vi "RT-PC Main.vi"() -> ()   [LabVIEW 2016]
panel:
  out "received message":string
  out "success":bool
  in  "[ESC]":bool
  in  "my name":string="name"
  in  "ping":bool
  in  "listening port":u16=50001
  in  "destination IP address":string
  out "my primary IP address":string
  out "my available IP addresses":string[](array[string])
  out "number of addresses":i32
  # "TCP ping"
  # "restart VI after changing\nlistening port number"
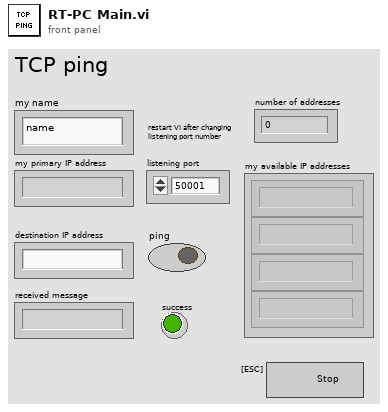
[diagram p1: front panel]
types:
  T1 = enum16{"Standard", "Buffered", "CRLF", "Immediate"}
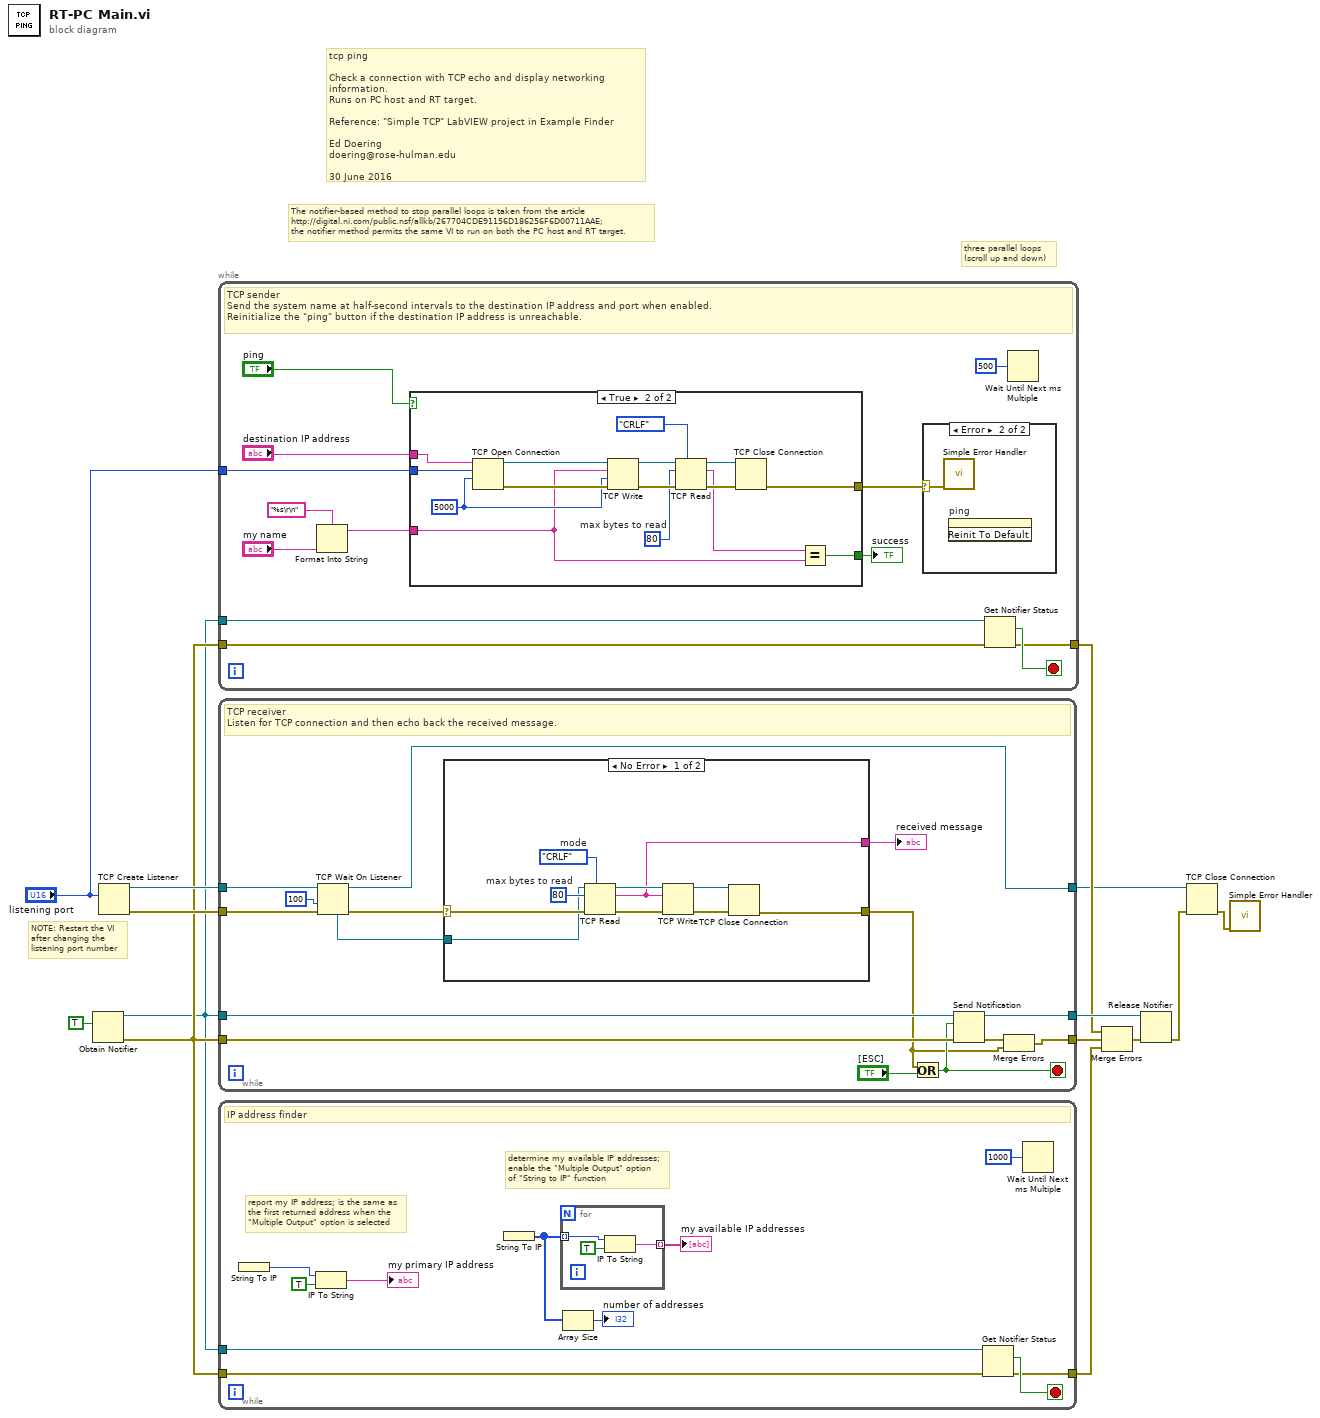
[diagram p0: block diagram]
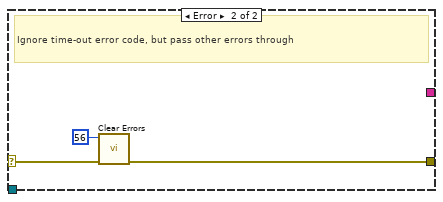
[diagram p2: hidden frame]
diagram:
  # "NOTE: Restart the VI\nafter changing the\nlistening port number"
  # "The notifier-based method to stop parallel loops is taken from the article\nhttp://digital.ni.com/public.nsf/allkb/267704CDE91156D186256F6D00711AAE;\nthe notifier method permits the same VI to run on both the PC host and RT target."
  # "three parallel loops\n(scroll up and down)"
  # "tcp ping\n\nCheck a connection with TCP echo and display networking information.\nRuns on PC host and RT target.\n\nReference: \"Simple TCP\" LabVIEW project in Example Finder \n\nEd Doering\ndoering@rose-hulman.edu\n\n30 June 2016"
  n1 = Obtain Notifier(notification data type=TRUE ("dot notation? (F)")) -> (notifier out=w4:refnum<notifier>, error out=w5:errorcluster)  [unwired: 3 in, 1 out]
  n2 = TCP Create Listener(10:"listening port") -> (0:w14:errorcluster, 3:w13:refnum<k5>)  [unwired: 4 in, 1 out]
  n3 = while {
    tunnel: w5 -> [w21]
    tunnel: w4 -> [w20]
    tunnel: [w18] -> w3
    tunnel: "listening port" -> [w15]
    stop <- w19 stop-if-true
    # "TCP sender\nSend the system name at half-second intervals to the destination IP address and port when enabled.\nReinitialize the \"ping\" button if the destination IP address is unreachable."
    n4 = Format Into String "Format Into String"(format string="%s\r\n", "my name") -> (resulting string=w24:string)  [unwired: 2 in, 1 out]
    n5 = case shown="True" "ping" {
      tunnel: [_ w33] -> w22
      tunnel: w24 -> [_ w32]
      tunnel: "destination IP address" -> [_ w43]
      tunnel: w15 -> [_ w42]
      tunnel: [_ w29] -> w16
      frame False {
      }
      frame True {
        w36 = 80  # max bytes to read
        w39 = 5000 ("timeout ms (60000)")
        n6 = TCP Open Connection(address=w43, remote port or service name=w42, timeout ms (60000)=w39) -> (connection ID=w40:refnum<k5>, error out=w41:errorcluster)  [unwired: 2 in]
        n7 = TCP Write(connection ID=w40, data in=w32, error in (no error)=w41, 9:w39) -> (connection ID out=w38:refnum<k5>, error out=w37:errorcluster)  [unwired: 1 out]
        n8 = TCP Read(connection ID=w38, bytes to read=w36, error in (no error)=w37, 7:T1."CRLF" ("mode (standard)")) -> (connection ID out=w34:refnum<k5>, data out=w30:string, error out=w35:errorcluster)  [unwired: 1 in]
        n9 = TCP Close Connection(connection ID=w34, error in (no error)=w35) -> (error out=w33:errorcluster)  [unwired: 1 in, 1 out]
        n10 = Equal?(x=w30, y=w32) -> (x = y?=w29:bool)
      }
    }
    "success" <- w16
    n11 = case shown="Error" w22 {
      selector: w22 -> [_ w28]
      frame No Error {
      }
      frame Error {
        n12 = call <vilib>:"Simple Error Handler.vi"("error in (no error)"=w28) -> ()  [unwired: 4 in, 5 out]
        n13 = invoke on="ping" class="Bool (strict)" method="Reinit To Default"() -> ()  [unwired: 3 in, 3 out]
      }
    }
    n14 = Get Notifier Status(notifier=w20, error in (no error)=w21) -> (current notification=w19:bool, error out=w18:errorcluster)  [unwired: 3 out]
    n15 = Wait Until Next ms Multiple(millisecond multiple=u32 500) -> ()  [unwired: 1 out]
  }
  n16 = while {
    tunnel: w13 -> [w58]
    tunnel: [w54] -> w1
    tunnel: w14 -> [w57]
    tunnel: w4 -> [w53]
    tunnel: w5 -> [w52]
    tunnel: [w46] -> w6
    tunnel: [w49] -> w11
    stop <- w50 stop-if-true
    # "TCP receiver\nListen for TCP connection and then echo back the received message."
    n17 = TCP Wait On Listener(8:w57, 9:100 ("timeout ms (25000)"), 11:w58) -> (0:w56:errorcluster, 3:w54:refnum<k5>, 4:w45:refnum<k5>)  [unwired: 1 in, 2 out]
    n18 = case shown="No Error" w56 {
      selector: w56 -> [w62 w71]
      tunnel: [w61 w70] -> w47
      tunnel: w45 -> [w60 _]
      tunnel: [w59 _] -> w44
      frame No Error {
        w64 = 80  # max bytes to read
        w63 = T1."CRLF"  # mode
        n19 = TCP Read(connection ID=w60, bytes to read=w64, error in (no error)=w62, 7:w63) -> (connection ID out=w66:refnum<k5>, data out=w59:string, error out=w68:errorcluster)  [unwired: 1 in]
        n20 = TCP Write(connection ID=w66, data in=w59, error in (no error)=w68) -> (connection ID out=w67:refnum<k5>, error out=w65:errorcluster)  [unwired: 1 in, 1 out]
        n21 = TCP Close Connection(connection ID=w67, error in (no error)=w65) -> (error out=w61:errorcluster)  [unwired: 1 in, 1 out]
      }
      frame Error {
        # "Ignore time-out error code, but pass other errors through"
        n22 = call <vilib>:"Clear Errors.vi"("error in (no error)"=w71, "specific error code to clear (0: all)"=56) -> ("error out"=w70:errorcluster)  [unwired: 4 in, 1 out]
      }
    }
    "received message" <- w44
    n23 = Or(x=w47, y="[ESC]") -> (x .or. y?=w50:bool)
    n24 = Send Notification(notification=w50, notifier=w53, error in (no error)=w52) -> (notifier out=w49:refnum<notifier>, error out=w48:errorcluster)
    n25 = Merge Errors(w48, w47) -> (w46:errorcluster)
  }
  n26 = while {
    tunnel: w5 -> [w75]
    tunnel: w4 -> [w74]
    tunnel: [w72] -> w10
    stop <- w73 stop-if-true
    # "determine my available IP addresses;\nenable the \"Multiple Output\" option\nof \"String to IP\" function"
    # "report my IP address; is the same as\nthe first returned address when the\n\"Multiple Output\" option is selected"
    # "IP address finder"
    n27 = String To IP() -> (0:w81:u32)  [unwired: 1 in]
    n28 = IP To String(1:TRUE ("dot notation? (F)"), 2:w81) -> (0:→"my primary IP address":string)
    n29 = String To IP() -> (0:w78:u32[])  [unwired: 1 in]
    n30 = for {
      tunnel: w78 -> [w84] mode=indexing
      tunnel: [w83] -> w79 mode=indexing
      n31 = IP To String(1:TRUE ("dot notation? (F)"), 2:w84) -> (0:w83:string)
    }
    "my available IP addresses" <- w79
    n32 = Array Size(array=w78) -> (size(s)=→"number of addresses":i32)
    n33 = Get Notifier Status(notifier=w74, error in (no error)=w75) -> (current notification=w73:bool, error out=w72:errorcluster)  [unwired: 3 out]
    n34 = Wait Until Next ms Multiple(millisecond multiple=u32 1000) -> ()  [unwired: 1 out]
  }
  n35 = Merge Errors(w3, w6, w10) -> (w9:errorcluster)
  n36 = Release Notifier(notifier=w11, error in (no error)=w9) -> (error out=w8:errorcluster)  [unwired: 1 in, 2 out]
  n37 = TCP Close Connection(connection ID=w1, error in (no error)=w8) -> (error out=w7:errorcluster)  [unwired: 1 in, 1 out]
  n38 = call <vilib>:"Simple Error Handler.vi"("error in (no error)"=w7) -> ()  [unwired: 4 in, 5 out]
